vi "Periodic Tasks.vi"(8 "error in":errorcluster) -> ()   [LabVIEW 2013]
doc: "This VI runs in parallel to other tasks. It can contain as many user-defined periodic loops as you need. These can carry out PID or other sorts of timed response."
uses:
  <vilib>/Rock Robotics/SystemInterfaces/Utilities/FPGA_UtilitiesLED Source.ctl
  <vilib>/Rock Robotics/SystemInterfaces/Utilities/FPGA_UtilitiesLED State.ctl
  <vilib>/Rock Robotics/WPI/Compressor/WPI_CompressorGetSetRefNum.vi
  Robot Global Data.vi
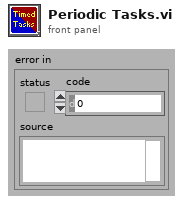
[diagram p1: front panel]
types:
  T1 = typedef "FPGA_UtilitiesLED State.ctl" = enum16{"Off", "On", "Toggle"}
  T2 = typedef "FPGA_UtilitiesLED Source.ctl" = enum16{"User LED", "FPGA LED"}
  T3 = typedef "TeleopInstruction.ctl" = cluster{"cDriveLeft":dbl, "cDriveRight":dbl, "cHalfDrive":bool, "cStraightDrive":bool, "cSonicShifter":bool}
  T4 = typedef "DriveQueueInstruction.ctl" = cluster{"DriveInstruction":T5, "Subsystem":T6, "DriveAction":T7, "LoopTiming":u32}
  T5 = typedef "DriveInstruction.ctl" = cluster{"cDriveLeft":dbl, "cDriveRight":dbl, "cHalfDrive":bool, "cStraightDrive":bool}
  T6 = typedef "QueueSubsystem.ctl" = enum16{"Drive", "Arm", "Catapult", "Roller"}
  T7 = typedef "DriveAction.ctl" = enum16{"Init", "LinearDrive", "SetValue", "Disable"}
  T8 = typedef "WPI_CompressorDevRef.ctl" = cluster{"DevStatus":errorcluster, "DigitalInputDevRef":T9, "RelayDevRef":T12}
  T9 = typedef "WPI_DigitalInputDevRef.ctl" = cluster{"DevStatus":errorcluster, "DIO Channel":T10, "Digital Module":T11}
  T10 = typedef "FPGA_DIOChannel.ctl" = enum8{"DIO 1", "DIO 2", "DIO 3", "DIO 4", "DIO 5", "DIO 6", "DIO 7", "DIO 8", "DIO 9", "DIO 10", "DIO 11", "DIO 12", "DIO 13", "DIO 14", "Invalid"}
  T11 = typedef "FPGA_TypedefDigitalModule.ctl" = enum16{"Digital Module 1", "Digital Module 2"}
  T12 = typedef "WPI_RelayDevRef.ctl" = cluster{"DevStatus":errorcluster, "Relay Channel":T13, "Digital Module":T11, "Relay Direction":T14}
  T13 = typedef "FPGA_DIORelayChannel.ctl" = enum8{"Relay 1", "Relay 2", "Relay 3", "Relay 4", "Relay 5", "Relay 6", "Relay 7", "Relay 8", "Invalid"}
  T14 = typedef "WPI_RelayDirection.ctl" = enum16{"Both directions", "Forward only", "Reverse only"}
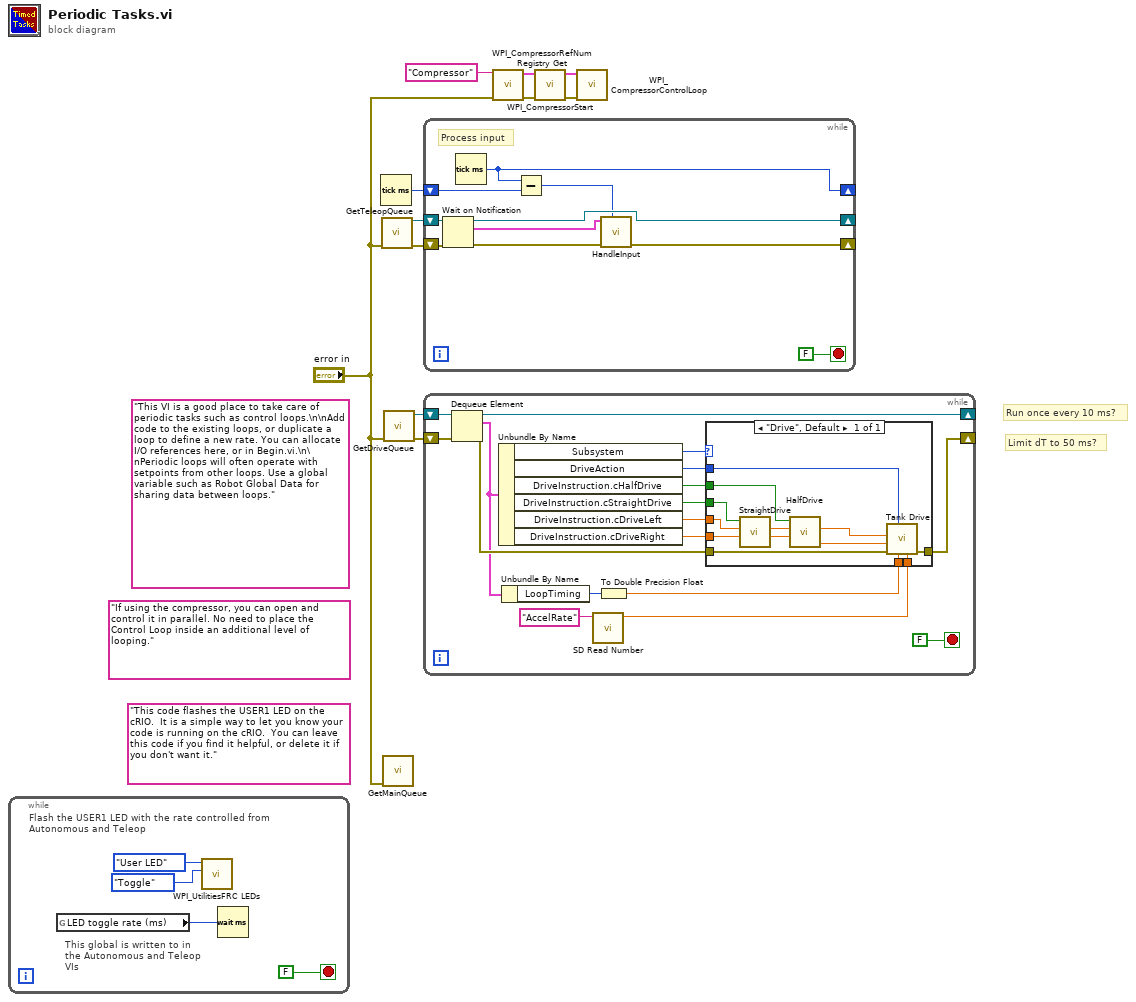
[diagram p0: block diagram]
diagram:
  (unwired) "If using the compressor, you can open and control it in parallel. No need to place the Control Loop inside an additional level of looping."
  (unwired) "This code flashes the USER1 LED on the cRIO.  It is a simple way to let you know your code is running on the cRIO.  You can leave this code if you find it helpful, or delete it if you don't want it."
  (unwired) "This VI is a good place to take care of periodic tasks such as control loops.\n\nAdd code to the existing loops, or duplicate a loop to define a new rate. You can allocate I/O references here, or in Begin.vi.\n\nPeriodic loops will often operate with setpoints from other loops. Use a global variable such as Robot Global Data for sharing data between loops."
  # "Limit dT to 50 ms?"
  # "Run once every 10 ms?"
  n1 = while {
    stop <- FALSE stop-if-true
    # "This global is written to in the Autonomous and Teleop VIs"
    # "Flash the USER1 LED with the rate controlled from Autonomous and Teleop"
    n2 = global read "Robot Global Data.vi" "LED toggle rate (ms)"() -> (w12:u32)
    n3 = call <vilib>:"WPI_UtilitiesFRC LEDs.vi"("State"=FPGA_UtilitiesLED_State."Toggle", "LED Type"=FPGA_UtilitiesLED_Source."User LED") -> ()  [unwired: 1 in, 9 out]
    n4 = Wait (ms)(milliseconds to wait=w12) -> ()  [unwired: 1 out]
  }
  n5 = Tick Count (ms)() -> (millisecond timer value=w1:u32)
  n6 = call "GetTeleopQueue.vi"("error in (no error)"="error in") -> ("error out"=w6:errorcluster, "notifier out"=w5:refnum<notifier>)  [unwired: 9 in]
  n7 = call "GetMainQueue.vi"("error in (no error)"="error in") -> ()  [unwired: 9 in, 2 out]
  n8 = call "GetDriveQueue.vi"("error in (no error)"="error in") -> ("error out"=w3:errorcluster, "queue out"=w2:refnum<queue>)  [unwired: 9 in]
  n9 = while {
    shift-right: [w22] -> _
    shift-left: w5 -> [w24]
    shift-right: [w20] -> _
    shift-left: w6 -> [w25]
    shift-right: [w18] -> _
    shift-left: w1 -> [w19]
    stop <- FALSE stop-if-true
    # "Process input"
    n10 = Wait on Notification(notifier=w24, error in (no error)=w25) -> (notifier out=w22:refnum<notifier>, notification=w17:T3, error out=w21:errorcluster)  [unwired: 2 in, 1 out]
    n11 = Tick Count (ms)() -> (millisecond timer value=w18:u32)
    n12 = Subtract(x=w18, y=w19) -> (x-y=w16:u32)
    n13 = call "HandleInput.vi"("LoopTiming"=w16, "error in (no error)"=w21, "TeleopInstruction"=w17) -> ("error out"=w20:errorcluster)  [unwired: 8 in]
  }
  n14 = while {
    shift-right: [w39] -> _
    shift-left: w3 -> [w41]
    shift-right: [w35] -> _
    shift-left: w2 -> [w36]
    stop <- FALSE stop-if-true
    n15 = Dequeue Element(queue=w36, error in (no error)=w41) -> (queue out=w35:refnum<queue>, element=w28:T4, error out=w40:errorcluster)  [unwired: 1 in, 1 out]
    n16 = Unbundle By Name(w28) -> ("Subsystem"=w34:T6, "DriveAction"=w33:T7, "DriveInstruction.cHalfDrive"=w32:bool, "DriveInstruction.cStraightDrive"=w31:bool, "DriveInstruction.cDriveLeft"=w30:dbl, "DriveInstruction.cDriveRight"=w29:dbl)
    n17 = Unbundle By Name(w28) -> ("LoopTiming"=w27:u32)
    n18 = call <vilib>:"SD Read Number.vi"("Name"="AccelRate") -> ("Numeric"=w37:dbl)  [unwired: 8 in, 2 out]
    n19 = To Double Precision Float(number=w27) -> (double precision float=w26:dbl)
    n20 = case shown="\"Drive\", Default" w34 {
      tunnel: w40 -> [w51]
      tunnel: [w50] -> w39
      tunnel: w37 -> [w49]
      tunnel: w33 -> [w48]
      tunnel: w32 -> [w46]
      tunnel: w31 -> [w47]
      tunnel: w30 -> [w45]
      tunnel: w29 -> [w44]
      tunnel: w26 -> [w43]
      frame "Drive", Default {
        n21 = call "StraightDrive.vi"("RightDrive in"=w44, "LeftDrive in"=w45, "StraightDrive"=w47) -> ("RightDrive out"=w54:dbl, "LeftDrive out"=w55:dbl)  [unwired: 7 in]
        n22 = call "HalfDrive.vi"("RightDrive in"=w54, "LeftDrive in"=w55, "HalfDrive"=w46) -> ("RightDrive out"=w52:dbl, "LeftDrive out"=w53:dbl)  [unwired: 7 in]
        n23 = call "Tank Drive.vi"("AccelRate"=w49, "LoopTime"=w43, "DriveAction"=w48, "error in (no error)"=w51, "RightDesired"=w52, "LeftDesired"=w53) -> ("error out"=w50:errorcluster)  [unwired: 5 in]
      }
    }
  }
  n24 = call <vilib>:"WPI_CompressorRefNum Registry Get.vi"("error in (no error)"="error in", "refnum name"="Compressor") -> ("error out"=w8:errorcluster, "CompressorDevRef"=w11:T8)  [unwired: 8 in]
  n25 = call <vilib>:"WPI_CompressorStart.vi"("error in (no error)"=w8, "CompressorDevRef"=w11) -> ("error out"=w7:errorcluster, "CompressorDevRef"=w10:T8)  [unwired: 8 in]
  n26 = call <vilib>:"WPI_CompressorControlLoop.vi"("error in (no error)"=w7, "CompressorDevRef"=w10) -> ()  [unwired: 10 in]
